vi "Check if specified tag is inside a Preset.vi"(8 "error in (no error)":errorcluster, 10 "Tag to check":string, 11 "Tree Refnum":refnum<vi>) -> (0 "error out":errorcluster, 1 "Specified Tag is a Preset command?":bool, 2 "Tag to add new item":string, 3 "Specified tag is part of a Preset?":bool)   [LabVIEW 2012]
doc: "SciScan 1.2 160622"
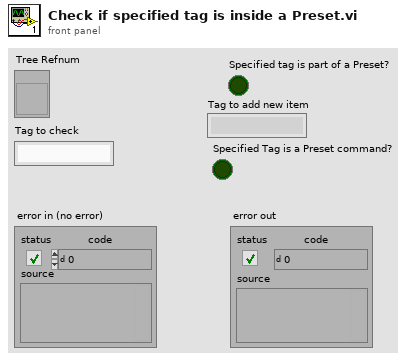
[diagram p1: front panel]
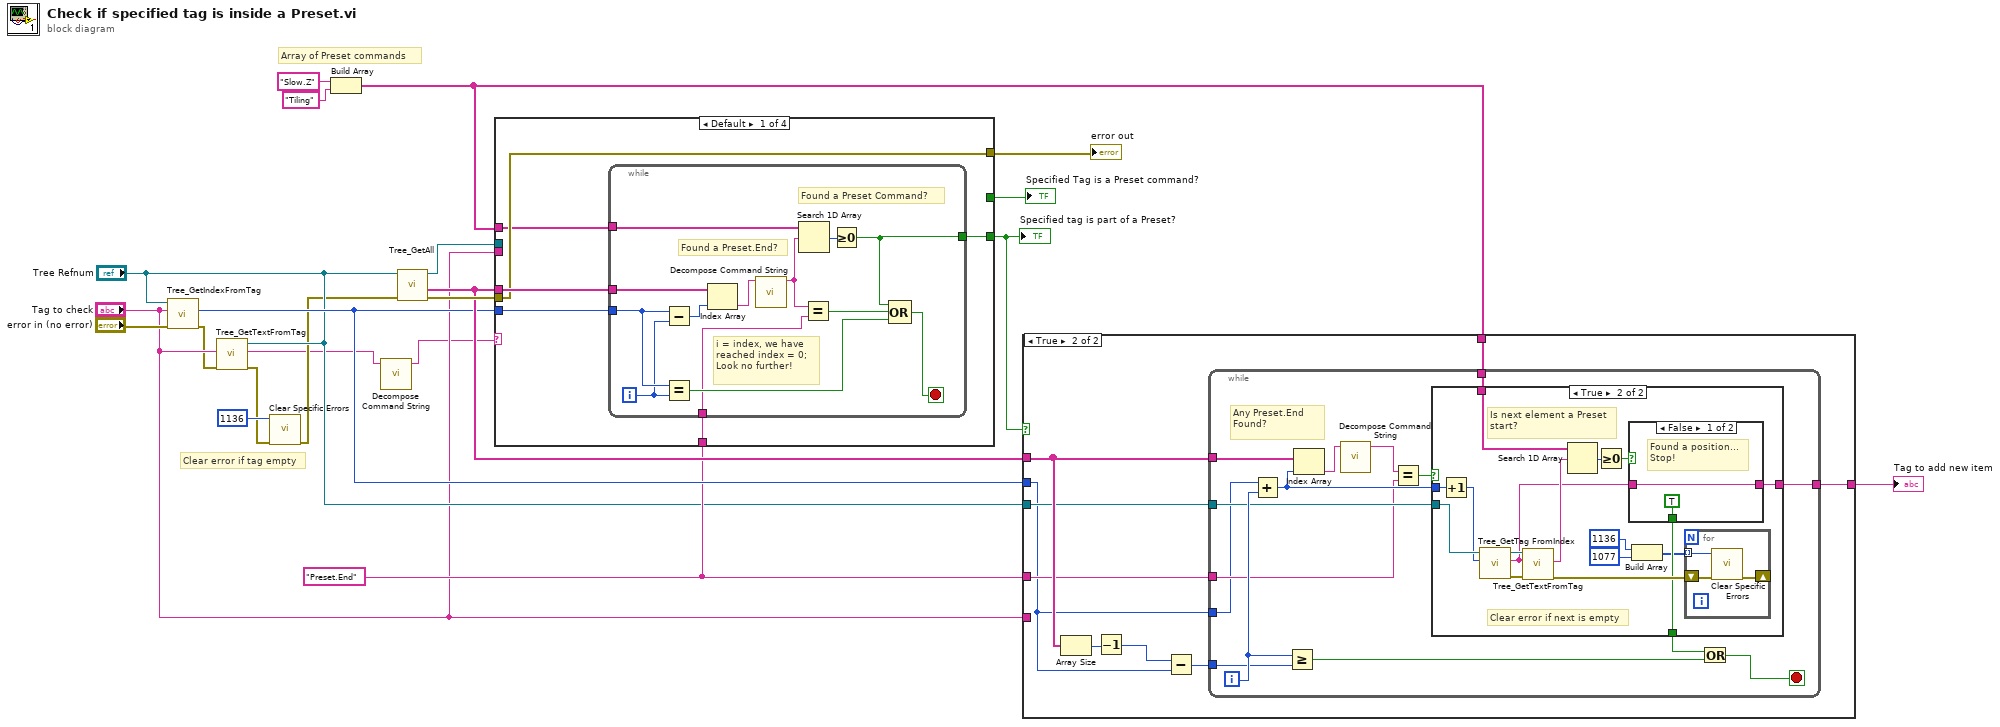
[diagram p0: block diagram]
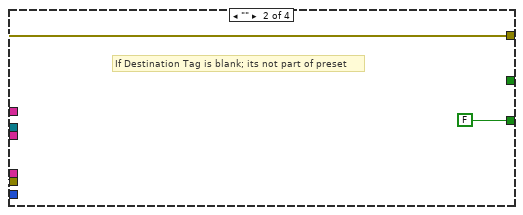
[diagram p5: hidden frame]
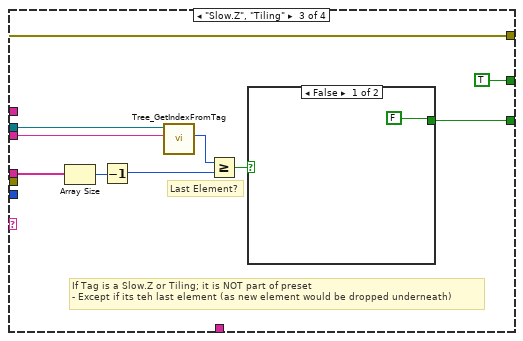
[diagram p6: hidden frame]
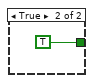
[diagram p7: hidden frame]
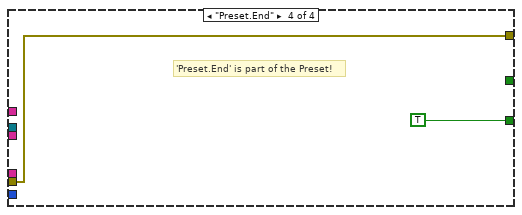
[diagram p8: hidden frame]
diagram:
  w11 = "Preset.End" ("y")
  # "Clear error if tag empty"
  # "Array of Preset commands"
  n1 = call "Tree_GetIndexFromTag.vi"("Error In"="error in (no error)", "Tag IN"="Tag to check", "Tree Refnum IN"="Tree Refnum") -> ("Error Out"=w6:errorcluster, "Index OUT"=w16:i32)  [unwired: 6 in, 1 out]
  n2 = call "Tree_GetTextFromTag.vi"("Error In"=w6, "Tag IN"="Tag to check", "Tree Refnum IN"="Tree Refnum") -> ("Error Out"=w5:errorcluster, "String OUT"=w2:string)  [unwired: 6 in, 1 out]
  n3 = call "Clear Specific Errors.vi"("Error In"=w5, "Error number In"=1136) -> ("Error Out"=w4:errorcluster)  [unwired: 8 in, 1 out]
  n4 = Build Array("Slow.Z" ("Tag to check"), "Tiling" ("Tag to check")) -> (w13:string[])
  n5 = call "Decompose Command String.vi"("Command IN"=w2) -> ("Action"=w1:string)  [unwired: 7 in, 3 out]
  n6 = call "Tree_GetAll.vi"("Error In"=w4, "Tree Refnum IN"="Tree Refnum") -> ("Error Out"=w18:errorcluster, "Text"=w17:string[], "Tree Refnum OUT"=w8:refnum<vi>)  [unwired: 6 in, 1 out]
  n7 = case shown="Default" w1 {
    tunnel: w18 -> [w24 w41 w52 w55]
    tunnel: [w27 FALSE w44 TRUE] -> w20
    tunnel: [w24 w41 w52 w55] -> w21
    tunnel: w17 -> [w26 _ w49 _]
    tunnel: w16 -> [w25 _ _ _]
    tunnel: w13 -> [w23 _ _ _]
    tunnel: w11 -> [w22 _ _ _]
    tunnel: w8 -> [_ _ w51 _]
    tunnel: "Tag to check" -> [_ _ w50 _]
    tunnel: [_ _ TRUE _] -> w3
    frame Default {
      n8 = while {
        tunnel: w26 -> [w38]
        tunnel: w23 -> [w36]
        tunnel: w25 -> [w40]
        tunnel: [w32] -> w27
        tunnel: w22 -> [w30]
        i -> [w39]
        stop <- w31 stop-if-true
        # "Found a Preset.End?"
        # "Found a Preset Command?"
        # "i = index, we have reached index = 0; Look no further!"
        n9 = Subtract(x=w40, y=w39) -> (x-y=w37:i32)
        n10 = Equal?(x=w40, y=w39) -> (x = y?=w34:bool)
        n11 = Index Array(array=w38, index=w37) -> (element=w29:string)
        n12 = call "Decompose Command String.vi"("Command IN"=w29) -> ("Action"=w28:string)  [unwired: 7 in, 3 out]
        n13 = Search 1D Array(1D array=w36, element=w28) -> (index of element=w35:i32)  [unwired: 1 in]
        n14 = Equal?(x=w28, y=w30) -> (x = y?=w33:bool)
        n15 = Greater Or Equal To 0?(x=w35) -> (x >= 0?=w32:bool)
        n16 = Compound Arithmetic op=OR(w32, w33, w34) -> (w31:bool)
      }
    }
    frame "" {
      # "If Destination Tag is blank; its not part of preset"
    }
    frame "Slow.Z", "Tiling" {
      # "Last Element?"
      # "If Tag is a Slow.Z or Tiling; it is NOT part of preset\n- Except if its teh last element (as new element would be dropped underneath)"
      n17 = Array Size(array=w49) -> (size(s)=w48:i32)
      n18 = Decrement(x=w48) -> (x-1=w46:i32)
      n19 = call "Tree_GetIndexFromTag.vi"("Tag IN"=w50, "Tree Refnum IN"=w51) -> ("Index OUT"=w47:i32)  [unwired: 7 in, 2 out]
      n20 = Greater Or Equal?(x=w47, y=w46) -> (x >= y?=w45:bool)
      n21 = case shown="False" w45 {
        tunnel: [FALSE TRUE] -> w44
        frame False {
        }
        frame True {
        }
      }
    }
    frame "Preset.End" {
      # "'Preset.End' is part of the Preset!"
    }
  }
  "error out" <- w21
  "Specified tag is part of a Preset?" <- w20
  "Specified Tag is a Preset command?" <- w3
  n22 = case shown="True" w20 {
    tunnel: w17 -> [_ w66]
    tunnel: w16 -> [_ w59]
    tunnel: "Tree Refnum" -> [_ w63]
    tunnel: w13 -> [_ w62]
    tunnel: [w57 w61] -> w12
    tunnel: "Tag to check" -> [w57 _]
    tunnel: w11 -> [_ w60]
    frame False {
      # "Specified tag is not part of a preset; hence its position can be used to add a preset."
    }
    frame True {
      n23 = Array Size(array=w66) -> (size(s)=w65:i32)
      n24 = Decrement(x=w65) -> (x-1=w58:i32)
      n25 = Subtract(x=w58, y=w59) -> (x-y=w64:i32)
      n26 = while {
        tunnel: w66 -> [w81]
        tunnel: w64 -> [w79]
        tunnel: w63 -> [w74]
        tunnel: w62 -> [w73]
        tunnel: [w71] -> w61
        tunnel: w60 -> [w70]
        tunnel: w59 -> [w69]
        i -> [w80]
        stop <- w77 stop-if-true
        # "Any Preset.End Found?"
        n27 = Add(x=w69, y=w80) -> (x+y=w75:i32)
        n28 = Greater Or Equal?(x=w80, y=w79) -> (x >= y?=w78:bool)
        n29 = Index Array(array=w81, index=w75) -> (element=w68:string)
        n30 = call "Decompose Command String.vi"("Command IN"=w68) -> ("Action"=w67:string)  [unwired: 7 in, 3 out]
        n31 = Equal?(x=w67, y=w70) -> (x = y?=w76:bool)
        n32 = case shown="True" w76 {
          tunnel: w75 -> [_ w97]
          tunnel: w74 -> [_ w96]
          tunnel: w73 -> [_ w94]
          tunnel: [_ w86] -> w72
          tunnel: [_ w89] -> w71
          frame False {
          }
          frame True {
            # "Clear error if next is empty"
            # "Is next element a Preset start?"
            n33 = Increment(x=w97) -> (x+1=w85:i32)
            n34 = call "Tree_GetTag FromIndex.vi"("Index IN"=w85, "Tree Refnum IN"=w96) -> ("Error Out"=w88:errorcluster, "Tag OUT"=w90:string, "Tree Refnum OUT"=w95:refnum<vi>)  [unwired: 7 in]
            n35 = call "Tree_GetTextFromTag.vi"("Error In"=w88, "Tag IN"=w90, "Tree Refnum IN"=w95) -> ("Error Out"=w87:errorcluster, "String OUT"=w93:string)  [unwired: 6 in, 1 out]
            n36 = Search 1D Array(1D array=w94, element=w93) -> (index of element=w92:i32)  [unwired: 1 in]
            n37 = Greater Or Equal To 0?(x=w92) -> (x >= 0?=w91:bool)
            n38 = case shown="False" w91 {
              tunnel: w90 -> [w102 _]
              tunnel: [w102 _] -> w89
              tunnel: [TRUE _] -> w86
              frame False {
                # "Found a position...\nStop!"
              }
              frame True {
              }
            }
            n39 = Build Array(1136 ("Error number In"), 1077 ("Error number In")) -> (w82:i32[])
            n40 = for {
              tunnel: w82 -> [w99] mode=indexing
              shift-right: [w98] -> _
              shift-left: w87 -> [w100]
              n41 = call "Clear Specific Errors.vi"("Error In"=w100, "Error number In"=w99) -> ("Error Out"=w98:errorcluster)  [unwired: 8 in, 1 out]
            }
          }
        }
        n42 = Or(x=w72, y=w78) -> (x .or. y?=w77:bool)
      }
    }
  }
  "Tag to add new item" <- w12
